vi "dvp Vi Get Analog Gain Descr.vi"(6 "pfDefault":sgl, 7 "pfMax":sgl, 9 "pfMin":sgl, 10 "pfStep":sgl, 11 "handle":u32) -> (1 "pfMin out":sgl, 2 "pfStep out":sgl, 3 "function return":u32(ring), 4 "pfDefault out":sgl, 5 "pfMax out":sgl)   [LabVIEW 2018, in "LabViewDVPCamera.lvlib"]
doc: "LabviewDvp2Api dvpStatus dvpViGetAnalogGainDescr(\n dvpHandle handle, \n float *pfStep,\n float *pfMin,\n float *pfMax,\n float *pfDefault\n);"
uses:
  LabViewDVPCamera.lvlib
  LabViewDVPCamera/LabViewDVPCamera.dll
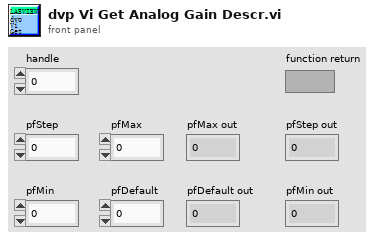
[diagram p1: front panel]
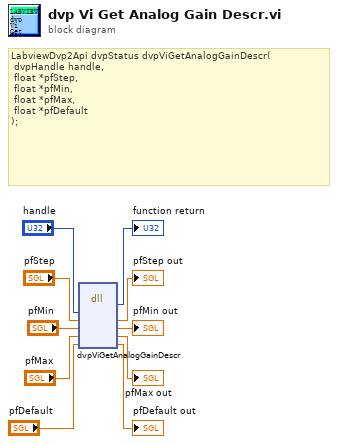
[diagram p0: block diagram]
diagram:
  # "LabviewDvp2Api dvpStatus dvpViGetAnalogGainDescr(\n\tdvpHandle handle, \n\tfloat *pfStep,\n\tfloat *pfMin,\n\tfloat *pfMax,\n\tfloat *pfDefault\n);"
  n1 = dll-call lib="C:/Program Files (x86)/DVP2 Labview cn 64/Sample/LabViewDVPCamera/LabViewDVPCamera.*" fn="dvpViGetAnalogGainDescr"("handle"="handle", "pfStep"="pfStep", "pfMin"="pfMin", "pfMax"="pfMax", "pfDefault"="pfDefault") -> (→"function return":u32, "pfStep"=→"pfStep out":sgl, "pfMin"=→"pfMin out":sgl, "pfMax"=→"pfMax out":sgl, "pfDefault"=→"pfDefault out":sgl)  [unwired: 4 in, 2 out]
